vi "EuniceF_Lab7 - Copy.vi"() -> ()   [LabVIEW 2025]
panel:
  out "Vtc,V":u8(slide) scale=0.0..5.0 scale format="%1.1f"
  out "TemperatureChart":dbl(graph)
  out "Vref,mV":dbl(slide) scale=0.0..5.0
  out "Vdiff,mV":dbl(slide) scale=0.0..2.0
  in  "STOP":bool
  out "Thermometer":dbl(slide) scale=-15.0..35.0
  out "Vscc,V":dbl(slide) scale=-10.0..10.0
  out "Heater":bool
  in  "Damping":dbl(slide) scale=0.0..10.0
  in  "Thermistor":dbl(slide) scale=0.0..100.0
  out "HIGH":bool
  out "LOW":bool
  out "Temperature, C":dbl(graph)
  out "Thermometer, C":dbl(slide) scale=0.0..100.0
  in  "stop":bool
  out "AtoD":i16 format="%x"
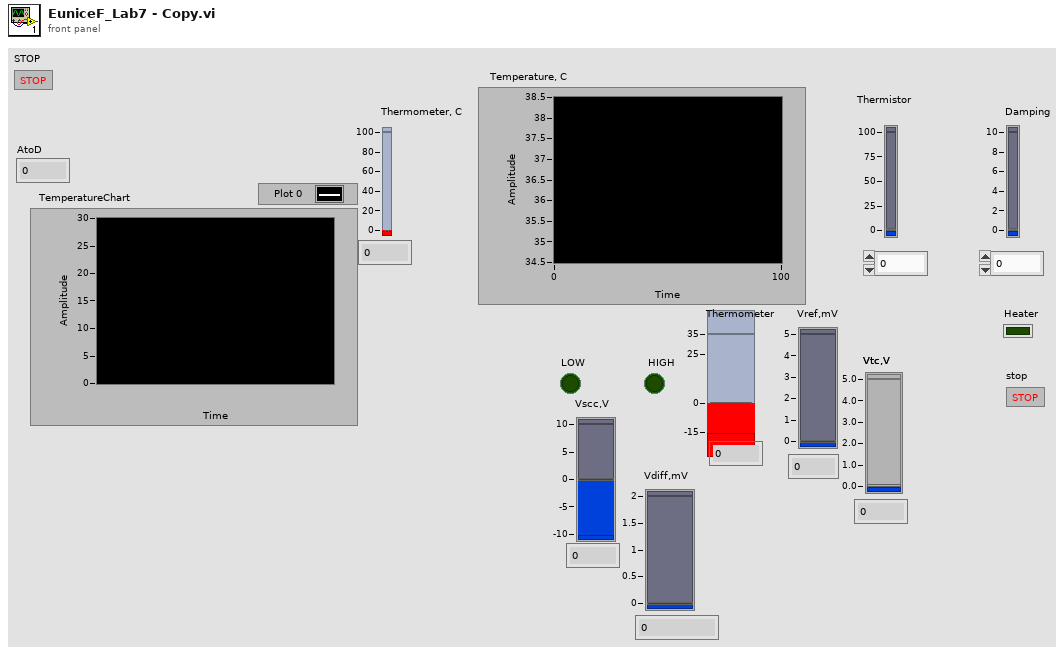
[diagram p1: front panel]
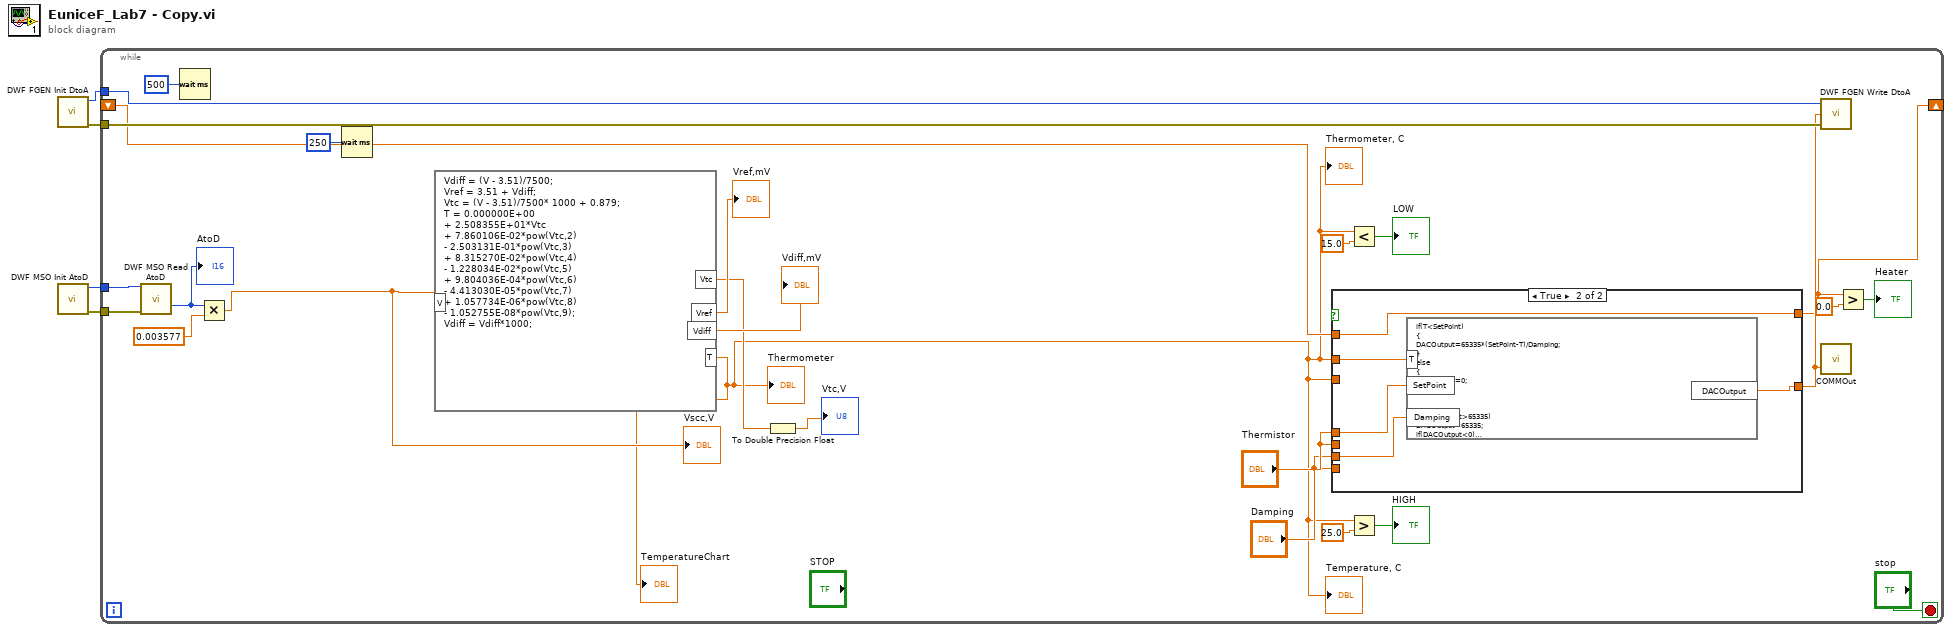
[diagram p0: block diagram]
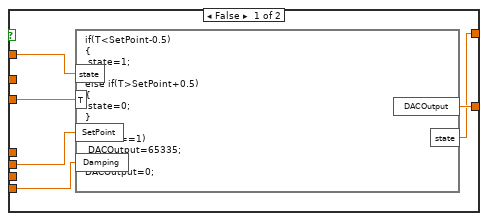
[diagram p2: hidden frame]
diagram:
  n1 = call "DWF FGEN Init DtoA.vi"() -> ("Error Out"=w1:errorcluster, "Instrument Handle Out"=w2:u32)  [unwired: 10 in]
  n2 = call "DWF MSO Init AtoD.vi"() -> ("Error Out"=w3:errorcluster, "Instrument Handle Out"=w4:i32)  [unwired: 10 in]
  n3 = while {
    tunnel: w4 -> [w30]
    tunnel: w3 -> [w29]
    shift-right: [w12] -> _
    shift-left: _ -> [w15]
    tunnel: w2 -> [w20]
    tunnel: w1 -> [w19]
    stop <- "stop" stop-if-true
    n4 = call "DWF MSO Read AtoD.vi"("Instrument Handle In AtoD"=w30, "Error In"=w29) -> ("AtoD"=w28:i16)  [unwired: 12 in, 1 out]
    "AtoD" <- w28
    n5 = Wait (ms)(milliseconds to wait=u32 500) -> ()  [unwired: 1 out]
    n6 = Multiply(x=w28, y=0.003577) -> (x*y=w6:dbl)
    "Vscc,V" <- w6
    n7 = Wait (ms)(milliseconds to wait=u32 250) -> ()  [unwired: 1 out]
    n8 = formula code="Vdiff = (V - 3.51)/7500;\nVref = 3.51 + Vdiff;\nVtc = (V - 3.51)/7500* 1000 + 0.879;\nT = 0.000000E+00\n+ 2.508355E+01*Vtc\n+ 7.860106E-02*pow(Vtc,2)\n- 2.503131E-01*pow(Vtc,3)\n+ 8.315270E-02*pow(Vtc,4)\n- 1.228034E-02*pow(Vtc,5)\n+ 9.804036E-04*pow(Vtc,6)\n- 4.413030E-05*pow(Vtc,7)\n+ 1.057734E-06*pow(Vtc,8)\n- 1.052755E-08*pow(Vtc,9);\nVdiff = Vdiff*1000;"("V"=w6) -> ("T"=w5:dbl, "Vdiff"=→"Vdiff,mV":dbl, "Vref"=→"Vref,mV":dbl, "Vtc"=w7:dbl)
    "Thermometer, C" <- w5
    "Temperature, C" <- w5
    "Thermometer" <- w5
    "TemperatureChart" <- w5
    n9 = To Double Precision Float(number=w7) -> (double precision float=→"Vtc,V":dbl)
    n10 = case shown="True" {
      selector: _ -> [_ _]
      tunnel: w5 -> [_ w41]
      tunnel: "Thermistor" -> [_ w40]
      tunnel: "Damping" -> [_ w39]
      tunnel: w5 -> [w36 _]
      tunnel: "Thermistor" -> [w35 _]
      tunnel: "Damping" -> [w34 _]
      tunnel: w15 -> [w33 w38]
      tunnel: [w32 w37] -> w14
      tunnel: [w31 w38] -> w12
      frame False {
        n11 = formula code="if(T<SetPoint-0.5)\n{\n state=1;\n}\nelse if(T>SetPoint+0.5)\n{ \n state=0;\n}\n\nif(state==1)\n DACOutput=65335;\nelse\nDACOutput=0;"("T"=w36, "SetPoint"=w35, "Damping"=w34, "state"=w33) -> ("DACOutput"=w32:dbl, "state"=w31:dbl)
      }
      frame True {
        n12 = formula code="if(T<SetPoint)\n{ \nDACOutput=65335*(SetPoint-T)/Damping;\n}\nelse\n{\nDACOutput=0;\n}\n\n\nif(DACOutput>65335)\nDACOutput=65335;\nif(DACOutput<0)\nDACOutput=0;"("T"=w41, "SetPoint"=w40, "Damping"=w39) -> ("DACOutput"=w37:dbl)
      }
    }
    n13 = Less?(x=w5, y=15.0) -> (x < y?=→"LOW":bool)
    n14 = Greater?(x=w5, y=25.0) -> (0:→"HIGH":bool)
    n15 = call "DWF FGEN Write DtoA.vi"("Error In"=w19, "Raw Data"=w14, "Instrument Handle In"=w20) -> ()  [unwired: 1 in, 2 out]
    n16 = call "COMMOut.vi"("Numeric"=w14) -> ()  [unwired: 1 in]
    n17 = Greater?(x=w12, y=0.0) -> (0:→"Heater":bool)
  }
